vi "ResMode.vi"() -> (0 "Resolution mode":enum16{"Single", "Double", "Quad"}(ring))   [LabVIEW 2017, in "GP22_TDC_Arduinoed.lvlib"]
doc: "Check the current state of the registers to see if autocal mode is enabled."
uses:
  GP22_TDC_Arduinoed.lvlib
  Public/Globals.vi
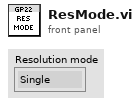
[diagram p1: front panel]
types:
  T1 = typedef "Registers.ctl" = cluster{"Reg0":u32, "Reg1":u32, "Reg2":u32, "Reg3":u32, "Reg4":u32, "Reg5":u32, "Reg6":u32}
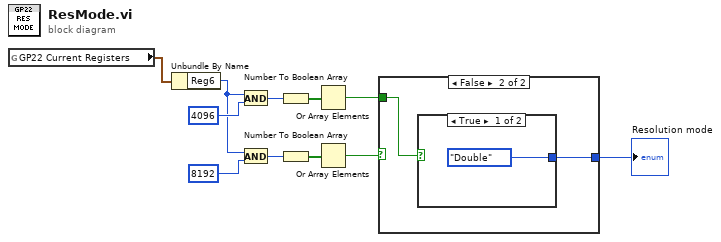
[diagram p0: block diagram]
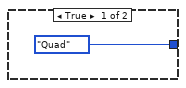
[diagram p2: hidden frame]
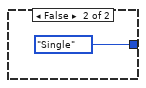
[diagram p3: hidden frame]
diagram:
  n1 = global read "Globals.vi" "GP22 Current Registers"() -> (w11:T1)
  n2 = Unbundle By Name(w11) -> ("Reg6"=w4:u32)
  n3 = And(x=w4, y=u32 4096 ("Reg0")) -> (x .and. y?=w9:u32)
  n4 = And(x=w4, y=u32 8192 ("Reg0")) -> (x .and. y?=w6:u32)
  n5 = Number To Boolean Array(number=w9) -> (Boolean array=w8:bool[])
  n6 = Number To Boolean Array(number=w6) -> (Boolean array=w5:bool[])
  n7 = Or Array Elements(Boolean array=w8) -> (logical OR=w1:bool)
  n8 = Or Array Elements(Boolean array=w5) -> (logical OR=w3:bool)
  n9 = case shown="False" w3 {
    tunnel: [enum16{"Single", "Double", "Quad"}."Quad" ("Resolution mode") w14] -> w2
    tunnel: w1 -> [_ w13]
    frame True {
    }
    frame False {
      n10 = case shown="True" w13 {
        tunnel: [enum16{"Single", "Double", "Quad"}."Double" ("Resolution mode") enum16{"Single", "Double", "Quad"}."Single" ("Resolution mode")] -> w14
        frame True {
        }
        frame False {
        }
      }
    }
  }
  "Resolution mode" <- w2
